vi "ni5660 Initialize.vi"(0 "downconverter device number":i16=1, 5 "digitizer resource name":string="DAQ::2", 7 "digitizer PLL lock time (sec)":dbl=1.0 min=0.0 format="%.2f", 9 "reset device":bool=TRUE, 11 "error in (no error)":errorcluster) -> (4 "receiver info out":T1, 15 "error out":errorcluster)   [LabVIEW 2011]
doc: "This VI performs the following initialization actions: \n\nCreates a new instrument driver session to the RF signal analyzer, using the downconverter device number and the digitizer resource name you specify \nSends initialization commands to reset both hardware modules to a known state necessary for NI-RFSA operation \nSets the RF downconverter module onboard clock as the RF Signal Analyzer reference clock source. When all the PLLs lock correctly, the STATUS light on the RF downconverter module is activated."
uses:
  <vilib>/addons/Modulation/niScope/controls/mod_Modulation Settings.ctl
  <instrlib>/niScope/Controls/niScope input clock source.ctl
  <instrlib>/niScope/Controls/niScope vertical coupling.ctl
  <vilib>/addons/Modulation/niScope/MT Initialize Receiver Info(RFSA).vi
  Instance          20 25Saved   ni5660 Initialize .vi
panel:
  in  "Case Constant\n(See Context Help)":bool=TRUE
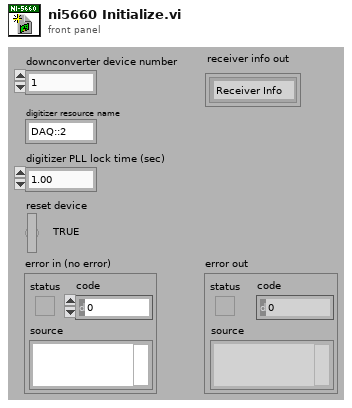
[diagram p1: front panel]
types:
  T1 = typedef "mod_Modulation Settings.ctl" = cluster{enum16{"Receiver Info"}, variant}
  T2 = typedef "niScope input clock source.ctl" = u16
  T3 = typedef "niScope vertical coupling.ctl" = i32
  T4 = typedef "mod_Writeable Attributes Cluster.ctl" = cluster{"receiver":cluster{"RFSA":cluster{"reference level":i32, "RF attenuation":i32}, "auto suppress SW IQ":enum16{"off", "on", "no change"}}}
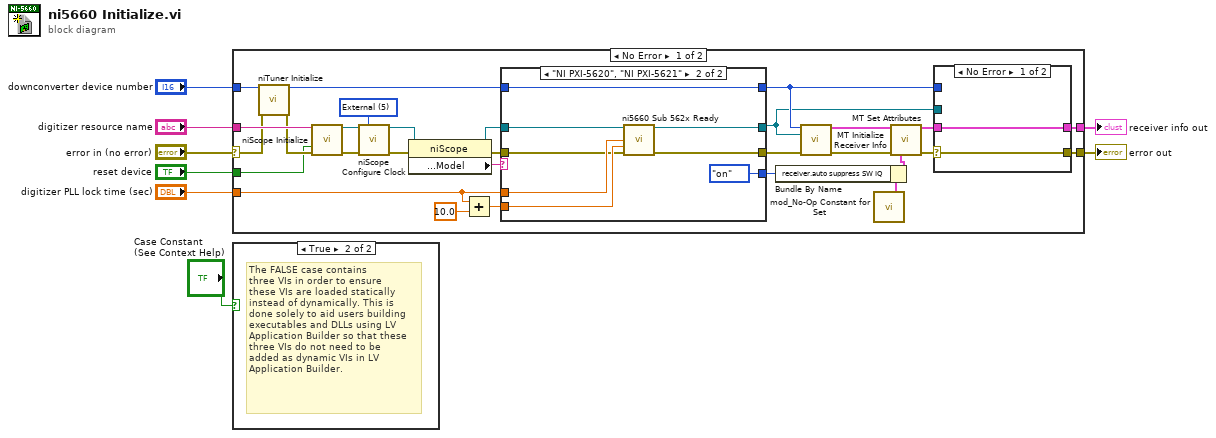
[diagram p0: block diagram]
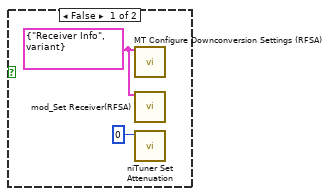
[diagram p2: hidden frame]
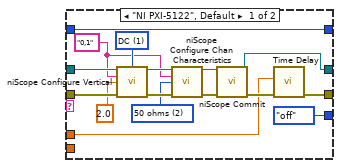
[diagram p3: hidden frame]
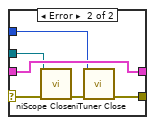
[diagram p4: hidden frame]
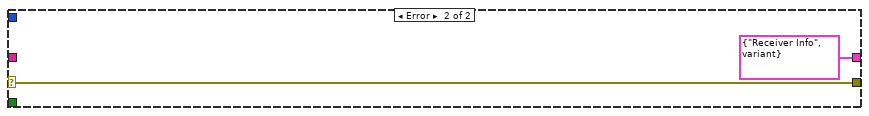
[diagram p5: hidden frame]
diagram:
  n1 = case shown="No Error" "error in (no error)" {
    selector: "error in (no error)" -> [w35 w71]
    tunnel: "digitizer resource name" -> [w37 _]
    tunnel: "downconverter device number" -> [w36 _]
    tunnel: "digitizer PLL lock time (sec)" -> [w28 _]
    tunnel: [w31 w71] -> w5
    tunnel: [w30 T1 {enum."Receiver Info", variant} ("receiver info out")] -> w3
    tunnel: "reset device" -> [w32 _]
    frame No Error {
      w29 = T2 5 items=["None"=0, "RTSI Clock"=1, "PFI 1"=2, "PFI 2"=3, "PXI Clock"=4, "External"=5, "Clock In"=7] ("input clock source")
      n2 = call <instrlib>:"niTuner Initialize.vi"("device number"=w36, "error in"=w35) -> ("taskID out"=w26:i32, "error out"=w34:errorcluster)  [unwired: 12 in]
      n3 = call <instrlib>:"niScope Initialize.vi"("resource name"=w37, "reset device"=w32, "error in"=w34) -> ("instrument handle"=w24:refnum<k15>, "error out"=w25:errorcluster)  [unwired: 11 in]
      n4 = call <instrlib>:"niScope Configure Clock.vi"("instrument handle"=w24, "input clock source"=w29, "error in"=w25) -> ("instrument handle out"=w21:refnum<k15>, "error out"=w23:errorcluster)  [unwired: 11 in]
      n5 = property class="niScope"(reference=w21, error in=w23) -> (reference out=w20:refnum<k15>, error out=w22:errorcluster, "Inherent IVI Attributes:Instrument Identification:Model"=w19:string)
      n6 = Add(x=w28, y=10.0) -> (x+y=w27:dbl)
      n7 = case shown="\"NI PXI-5620\", \"NI PXI-5621\"" w19 {
        tunnel: [w41 w55] -> w12
        tunnel: w28 -> [w39 w61]
        tunnel: w27 -> [_ w60]
        tunnel: [w40 w59] -> w13
        tunnel: w26 -> [w47 w56]
        tunnel: w22 -> [w52 w58]
        tunnel: w20 -> [w53 w57]
        tunnel: [w47 w56] -> w14
        tunnel: [enum16{"off", "on", "no change"}."off" ("receiver.auto suppress SW IQ") enum16{"off", "on", "no change"}."on" ("receiver.auto suppress SW IQ")] -> w11
        frame "NI PXI-5122", Default {
          w46 = u32 2 items=["1 mega ohm"=0, "50 ohms"=2] ("input impedance")
          w50 = T3 1 items=["AC", "DC", "Ground"] ("vertical coupling")
          w38 = "0,1" ("channel name")
          n8 = call <instrlib>:"niScope Configure Vertical.vi"("instrument handle"=w53, "vertical coupling"=w50, "channels"=w38, "vertical range"=2.0, "error in"=w52) -> ("instrument handle out"=w49:refnum<k15>, "error out"=w48:errorcluster)  [unwired: 9 in]
          n9 = call <instrlib>:"niScope Configure Chan Characteristics.vi"("instrument handle"=w49, "channels"=w38, "input impedance"=w46, "error in"=w48) -> ("instrument handle out"=w44:refnum<k15>, "error out"=w43:errorcluster)  [unwired: 10 in]
          n10 = call <instrlib>:"niScope Commit.vi"("instrument handle"=w44, "error in"=w43) -> ("instrument handle out"=w40:refnum<k15>, "error out"=w42:errorcluster)  [unwired: 12 in]
          n11 = call "Time Delay"("error in (no error)"=w42, "Delay Time (s)"=w39) -> ("error out"=w41:errorcluster)  [unwired: 9 in]
        }
        frame "NI PXI-5620", "NI PXI-5621" {
          n12 = call <instrlib>:"ni5660 Sub 562x Ready.vi"("instrument handle in"=w57, "PLL lock time (sec)"=w61, "max timeout (sec)"=w60, "error in (no error)"=w58) -> ("instrument handle out"=w59:refnum<k15>, "error out"=w55:errorcluster)  [unwired: 10 in]
        }
      }
      n13 = call-poly <vilib>:"MT Initialize Receiver Info.vi"("niTuner taskID"=w14, "niScope handle"=w13, "error in (no error)"=w12) -> ("receiver info out"=w15:T1, "error out"=w16:errorcluster)  [unwired: 11 in]
      n14 = call <vilib>:"mod_No-Op Constant for Set.vi"() -> ("no-op parameters"=w17:T4)
      n15 = Bundle By Name(cluster=w17, "receiver.auto suppress SW IQ"=w11) -> (w18:T4)
      n16 = call <vilib>:"MT Set Attributes.vi"("receiver info in"=w15, "error in (no error)"=w16, "attributes"=w18) -> ("receiver info out"=w10:T1, "error out"=w9:errorcluster)  [unwired: 11 in]
      n17 = case shown="No Error" w9 {
        selector: w9 -> [w62 w68]
        tunnel: [w63 w69] -> w30
        tunnel: w10 -> [w63 w69]
        tunnel: w13 -> [_ w64]
        tunnel: [w62 w66] -> w31
        tunnel: w14 -> [_ w65]
        frame No Error {
        }
        frame Error {
          n18 = call <instrlib>:"niScope Close.vi"("instrument handle"=w64, "error in"=w68) -> ("error out"=w67:errorcluster)  [unwired: 13 in]
          n19 = call <instrlib>:"niTuner Close.vi"("error in"=w67, "taskID in"=w65) -> ("error out"=w66:errorcluster)  [unwired: 9 in]
        }
      }
    }
    frame Error {
    }
  }
  "error out" <- w5
  "receiver info out" <- w3
  n20 = case shown="True" "Case Constant\n(See Context Help)" {
    frame False {
      w72 = T1 {enum."Receiver Info", variant} ("receiver info in")
      n21 = call <vilib>:"MT Configure Downconversion Settings (RFSA).vi"("receiver info in"=w72) -> ()  [unwired: 11 in, 4 out]
      n22 = call <vilib>:"mod_Set Receiver(RFSA).vi"("receiver info in"=w72) -> ()  [unwired: 13 in, 2 out]
      n23 = call <instrlib>:"niTuner Set Attenuation.vi"("taskID in"=0) -> ()  [unwired: 7 in, 4 out]
    }
    frame True {
      # "The FALSE case contains\nthree VIs in order to ensure\nthese VIs are loaded statically\ninstead of dynamically. This is\ndone solely to aid users building\nexecutables and DLLs using LV\nApplication Builder so that these\nthree VIs do not need to be\nadded as dynamic VIs in LV\nApplication Builder."
    }
  }
